vi "Get Measruement Scenario.vi"(11 "Measurement properties":T1={"Measurement ID"=enum."1 signal, 1 ADC, 1 PJVS", "Description"="3 phase, 3 ADC, 1 PJVS", "Switching matrix M"=[], "Signal frequency  (Hz)"=50.0, "Maximal signal amplitude (V)"=0.0, "PRs (s)"=1.0, "PRe (s)"=50.0, "MRs (s)"=0.0, "MRe (s)"=0.0, "Set PJVS frequency (Hz)"=50.0, "PJVS reference voltages (1 period, V)"=[], "Requiested PJVS steps"=10, "Sampling f (Hz)"=0.0, "Trigger mode"=enum."Trigger every MX switch", "Timing matrix (periods)"=[], "Record length (multiples of M)"=1, "Calculated"={"Triggers to next path (line of sequence)"=[], "Record samples"=0, "Sample indexes of switches"=[], "PRs (samples)"=0, "PRe (samples)"=0, "MRs (samples)"=0, "MRe (samples)"=0, "Trigger frequency  (Hz)"=50.0, "Measurement druation (s)"=0.0, "Samples per step"=0.0, "QPMX Sequence"=[]}, "No of required digitizers"=0, "No of required transducers"=0, "Transducer correction files"=[], "Digitizer correction file"=path ""} {"Calculated"."Trigger frequency  (Hz)" format="%#_6p"; "Record length (multiples of M)" min=1 step=1; "PJVS reference voltages (1 period, V)" format="%.9g"; "MRe (s)" format="%#_4p"; "MRs (s)" format="%#_4p"; "PRe (s)" format="%#.4p"; "PRs (s)" format="%#_4p"}) -> (3 "Measurement properties out":T1={"Measurement ID"=enum."1 signal, 1 ADC, 1 PJVS", "Description"="3 phase, 3 ADC, 1 PJVS", "Switching matrix M"=[], "Signal frequency  (Hz)"=50.0, "Maximal signal amplitude (V)"=0.0, "PRs (s)"=1.0, "PRe (s)"=50.0, "MRs (s)"=0.0, "MRe (s)"=0.0, "Set PJVS frequency (Hz)"=50.0, "PJVS reference voltages (1 period, V)"=[], "Requiested PJVS steps"=10, "Sampling f (Hz)"=0.0, "Trigger mode"=enum."Trigger every MX switch", "Timing matrix (periods)"=[], "Record length (multiples of M)"=1, "Calculated"={"Triggers to next path (line of sequence)"=[], "Record samples"=0, "Sample indexes of switches"=[], "PRs (samples)"=0, "PRe (samples)"=0, "MRs (samples)"=0, "MRe (samples)"=0, "Trigger frequency  (Hz)"=50.0, "Measurement druation (s)"=0.0, "Samples per step"=0.0, "QPMX Sequence"=[]}, "No of required digitizers"=0, "No of required transducers"=0, "Transducer correction files"=[], "Digitizer correction file"=path ""} {"Calculated"."Trigger frequency  (Hz)" format="%#_6p"; "Record length (multiples of M)" min=1 step=1; "PJVS reference voltages (1 period, V)" format="%.9g"; "MRe (s)" format="%#_4p"; "MRs (s)" format="%#_4p"; "PRe (s)" format="%#.4p"; "PRs (s)" format="%#_4p"})   [LabVIEW 2020]
doc: "Based on the Measurement scenario ID, VI generates Switching matrix M, Timing matrix and QPMX Sequence."
uses:
  Type definitions/Measuement properties.ctl
  Type definitions/Measurement ID.ctl
  Type definitions/Trigger mode.ctl
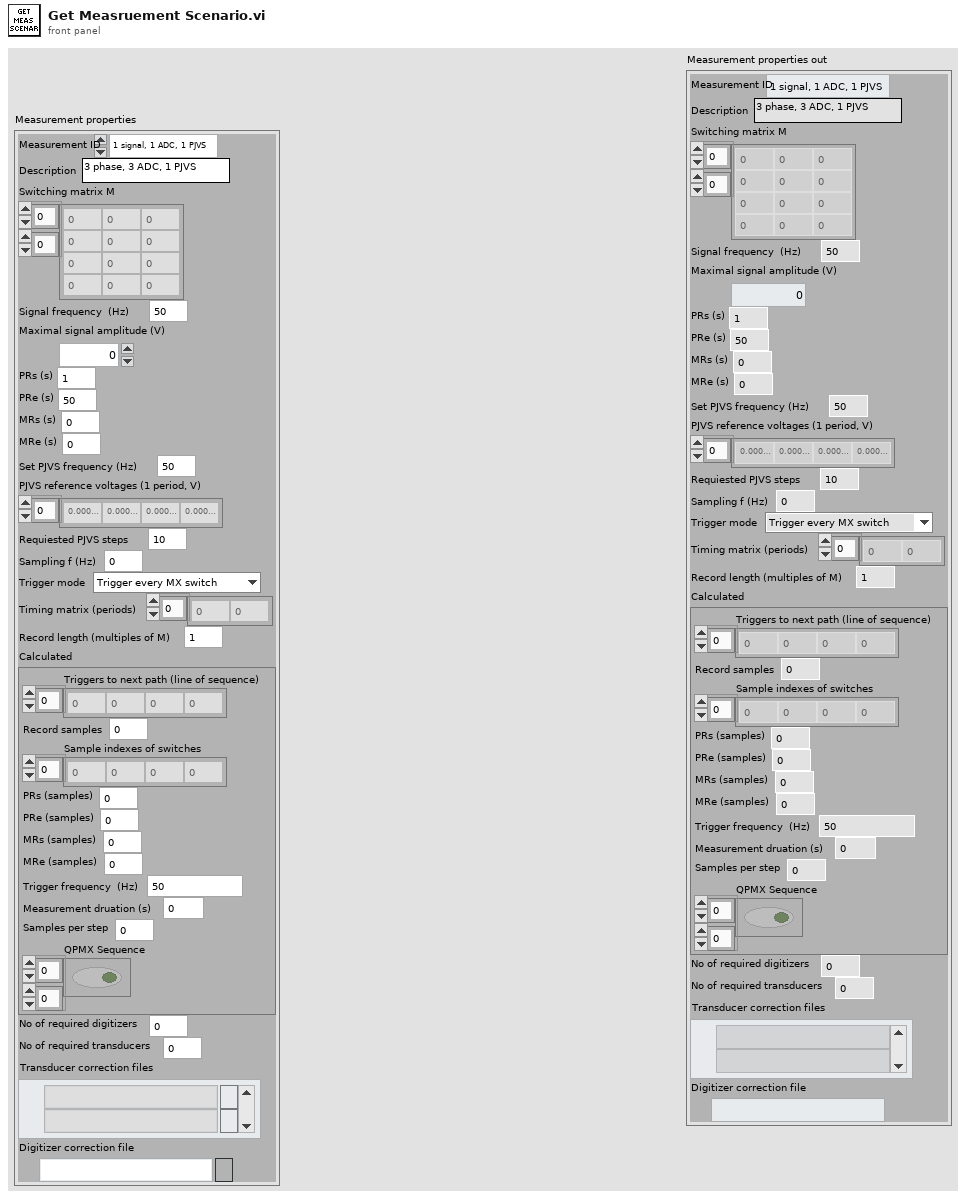
[diagram p1: front panel]
types:
  T1 = typedef "Measuement properties.ctl" = cluster{"Measurement ID":T2, "Description":string, "Switching matrix M":i32[][], "Signal frequency  (Hz)":dbl, "Maximal signal amplitude (V)":dbl, "PRs (s)":dbl, "PRe (s)":dbl, "MRs (s)":dbl, "MRe (s)":dbl, "Set PJVS frequency (Hz)":dbl, "PJVS reference voltages (1 period, V)":dbl[], "Requiested PJVS steps":u32, "Sampling f (Hz)":dbl, "Trigger mode":T3, "Timing matrix (periods)":i32[], "Record length (multiples of M)":u32, "Calculated":cluster{"Triggers to next path (line of sequence)":u32[], "Record samples":u32, "Sample indexes of switches":u32[], "PRs (samples)":i32, "PRe (samples)":i32, "MRs (samples)":i32, "MRe (samples)":i32, "Trigger frequency  (Hz)":dbl, "Measurement druation (s)":dbl, "Samples per step":dbl, "QPMX Sequence":bool[][]}, "No of required digitizers":u32, "No of required transducers":u32, "Transducer correction files":path[], "Digitizer correction file":path}
  T2 = typedef "Measurement ID.ctl" = enum16{"Manual setup", "1 signal, 1 ADC, 1 PJVS", "1 phase (U, I), 1 ADC, 1 PJVS", "1 phase (U, I), 2 ADC, 1 PJVS", "1 phase (U, I), 3 ADC, 1 PJVS", "3 phases (U1..3, I1..3), 3 ADC, 1 PJVS"}
  T3 = typedef "Trigger mode.ctl" = enum16{"Trigger every MX switch", "Trigger every sample"}
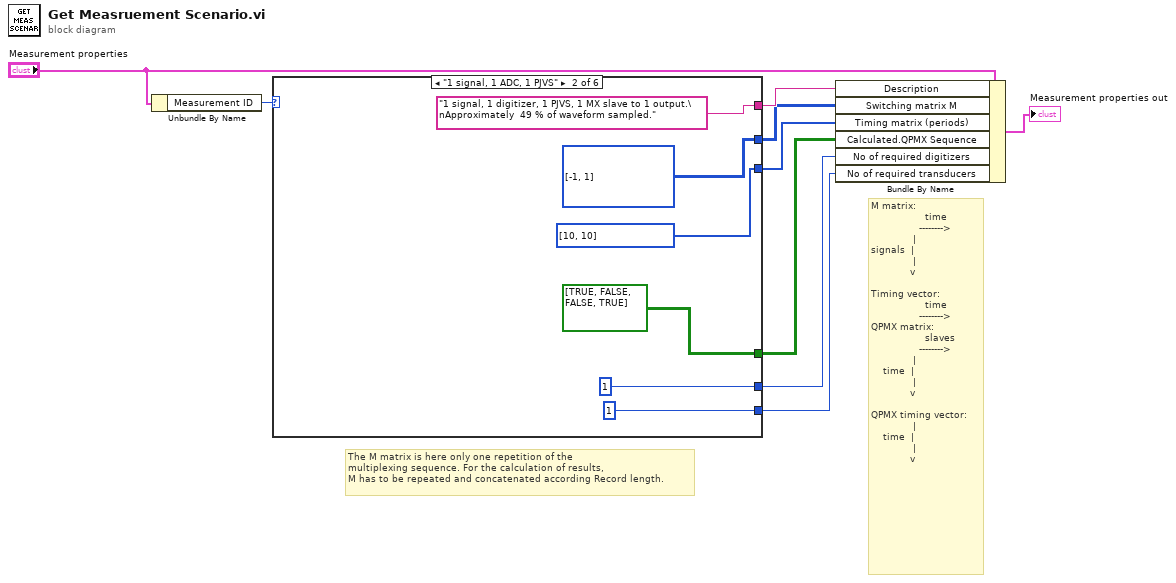
[diagram p0: block diagram]
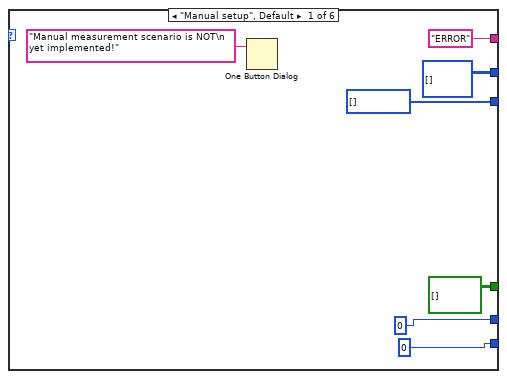
[diagram p2: hidden frame]
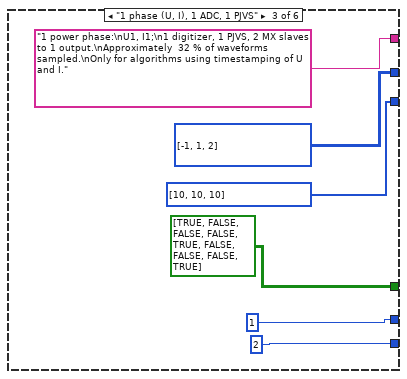
[diagram p3: hidden frame]
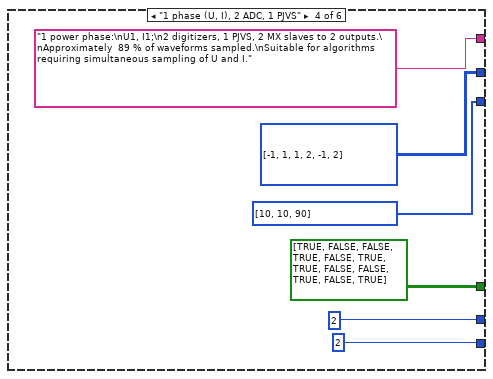
[diagram p4: hidden frame]
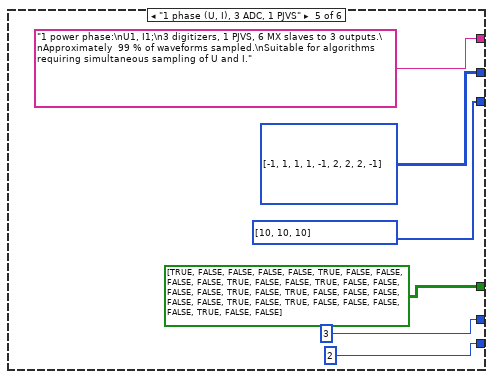
[diagram p5: hidden frame]
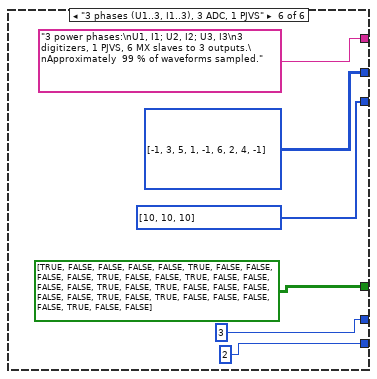
[diagram p6: hidden frame]
diagram:
  # "The M matrix is here only one repetition of the\nmultiplexing sequence. For the calculation of results,\nM has to be repeated and concatenated according Record length."
  # "M matrix:\n                  time\n                -------->\n              |\nsignals  |\n              | \n             v\n\nTiming vector:\n                  time\n                -------->\nQPMX matrix:\n                  slaves\n                -------->\n              |\n    time  |\n              | \n             v\n\nQPMX timing vector:\n              |\n    time  |\n              | \n             v"
  n1 = Unbundle By Name("Measurement properties") -> ("Measurement ID"=w7:T2)
  n2 = case shown="\"1 signal, 1 ADC, 1 PJVS\"" w7 {
    tunnel: ["ERROR" "1 signal, 1 digitizer, 1 PJVS, 1 MX slave to 1 output.\nApproximately  49 % of waveform sampled." "1 power phase:\nU1, I1;\n1 digitizer, 1 PJVS, 2 MX slaves to 1 output.\nApproximately  32 % of waveforms sampled.\nOnly for algorithms using timestamping of U and I." "1 power phase:\nU1, I1;\n2 digitizers, 1 PJVS, 2 MX slaves to 2 outputs.\nApproximately  89 % of waveforms sampled.\nSuitable for algorithms requiring simultaneous sampling of U and I." "1 power phase:\nU1, I1;\n3 digitizers, 1 PJVS, 6 MX slaves to 3 outputs.\nApproximately  99 % of waveforms sampled.\nSuitable for algorithms requiring simultaneous sampling of U and I." "3 power phases:\nU1, I1; U2, I2; U3, I3\n3 digitizers, 1 PJVS, 6 MX slaves to 3 outputs.\nApproximately  99 % of waveforms sampled."] -> w9
    tunnel: [i32[][] [] ("M") i32[][] [[-1, 1]] ("M") i32[][] [[-1, 1, 2]] ("M") i32[][] [[-1, 1, 1], [2, -1, 2]] ("M") i32[][] [[-1, 1, 1], [1, -1, 2], [2, 2, -1]] ("M") i32[][] [[-1, 3, 5], [1, -1, 6], [2, 4, -1]] ("M")] -> w8
    tunnel: [i32[] [] ("Timing matrix (periods)") i32[] [10, 10] ("Timing matrix (periods)") i32[] [10, 10, 10] ("Timing matrix (periods)") i32[] [10, 10, 90] ("Timing matrix (periods)") i32[] [10, 10, 10] ("Timing matrix (periods)") i32[] [10, 10, 10] ("Timing matrix (periods)")] -> w6
    tunnel: [bool[][] [] ("M") bool[][] [[TRUE, FALSE], [FALSE, TRUE]] ("M") bool[][] [[TRUE, FALSE, FALSE], [FALSE, TRUE, FALSE], [FALSE, FALSE, TRUE]] ("M") bool[][] [[TRUE, FALSE, FALSE, TRUE], [FALSE, TRUE, TRUE, FALSE], [FALSE, TRUE, FALSE, TRUE]] ("M") bool[][] [[TRUE, FALSE, FALSE, FALSE, FALSE, TRUE, FALSE, FALSE, FALSE, FALSE, TRUE, FALSE], [FALSE, TRUE, FALSE, FALSE, FALSE, FALSE, TRUE, FALSE, TRUE, FALSE, FALSE, FALSE], [FALSE, FALSE, TRUE, FALSE, TRUE, FALSE, FALSE, FALSE, FALSE, TRUE, FALSE, FALSE]] ("M") bool[][] [[TRUE, FALSE, FALSE, FALSE, FALSE, TRUE, FALSE, FALSE, FALSE, FALSE, TRUE, FALSE], [FALSE, TRUE, FALSE, FALSE, FALSE, FALSE, TRUE, FALSE, TRUE, FALSE, FALSE, FALSE], [FALSE, FALSE, TRUE, FALSE, TRUE, FALSE, FALSE, FALSE, FALSE, TRUE, FALSE, FALSE]] ("M")] -> w3
    tunnel: [u32 0 ("No of digitizers") u32 1 ("No of digitizers") u32 1 ("No of digitizers") u32 2 ("No of digitizers") u32 3 ("No of digitizers") u32 3 ("No of digitizers")] -> w2
    tunnel: [u32 0 ("No of digitizers") u32 1 ("No of digitizers") u32 2 ("No of digitizers") u32 2 ("No of digitizers") u32 2 ("No of digitizers") u32 2 ("No of digitizers")] -> w1
    frame "Manual setup", Default {
      n3 = One Button Dialog(message="Manual measurement scenario is NOT\n yet implemented!") -> ()  [unwired: 1 in, 1 out]
    }
    frame "1 signal, 1 ADC, 1 PJVS" {
    }
    frame "1 phase (U, I), 1 ADC, 1 PJVS" {
    }
    frame "1 phase (U, I), 2 ADC, 1 PJVS" {
    }
    frame "1 phase (U, I), 3 ADC, 1 PJVS" {
      (unwired) bool[][] [[TRUE, FALSE, FALSE, FALSE, FALSE, TRUE, FALSE, FALSE, FALSE, FALSE, TRUE, FALSE], [FALSE, TRUE, FALSE, FALSE, FALSE, FALSE, TRUE, FALSE, TRUE, FALSE, FALSE, FALSE], [FALSE, FALSE, TRUE, FALSE, TRUE, FALSE, FALSE, FALSE, FALSE, TRUE, FALSE, FALSE]] ("M")
    }
    frame "3 phases (U1..3, I1..3), 3 ADC, 1 PJVS" {
    }
  }
  n4 = Bundle By Name(cluster="Measurement properties", "Description"=w9, "Switching matrix M"=w8, "Timing matrix (periods)"=w6, "Calculated.QPMX Sequence"=w3, "No of required digitizers"=w2, "No of required transducers"=w1) -> (→"Measurement properties out":T1)
